vi "processamento_temperatura_velocidade.vi"() -> ()   [LabVIEW 2018]
uses:
  <vilib>/Analysis/NI_AALBase.lvlib
panel:
  in  "Velocidade":path
  out "Velocidade média":dbl format="%0.2f"
  out "Desvio-padrão da temperatura":dbl format="%0.2f"
  out "Temperatura Média":dbl format="%0.2f"
  out "x/y 2":dbl[](array[numeric])
  out "x-y 2":dbl
  out "direito 3":dbl
  out "esquerdo 3":dbl
  in  "Frequência de amostragem - velocidade":dbl
  out "Velocidade":waveform(dbl)(graph)
  out "x/y":dbl[](array[numeric])
  out "x-y":dbl
  out "direito 2":dbl
  out "esquerdo 2":dbl
  in  "Frequência de amostragem - temperatura":dbl
  out "Temperatura":waveform(dbl)(graph)
  in  "stop":bool
  in  "Temperatura":path
  # "PROGRAMA PARA O PROCESSAMENTO CONJUNTO \nDA TEMPERATURA E DA VELOCIDADE"
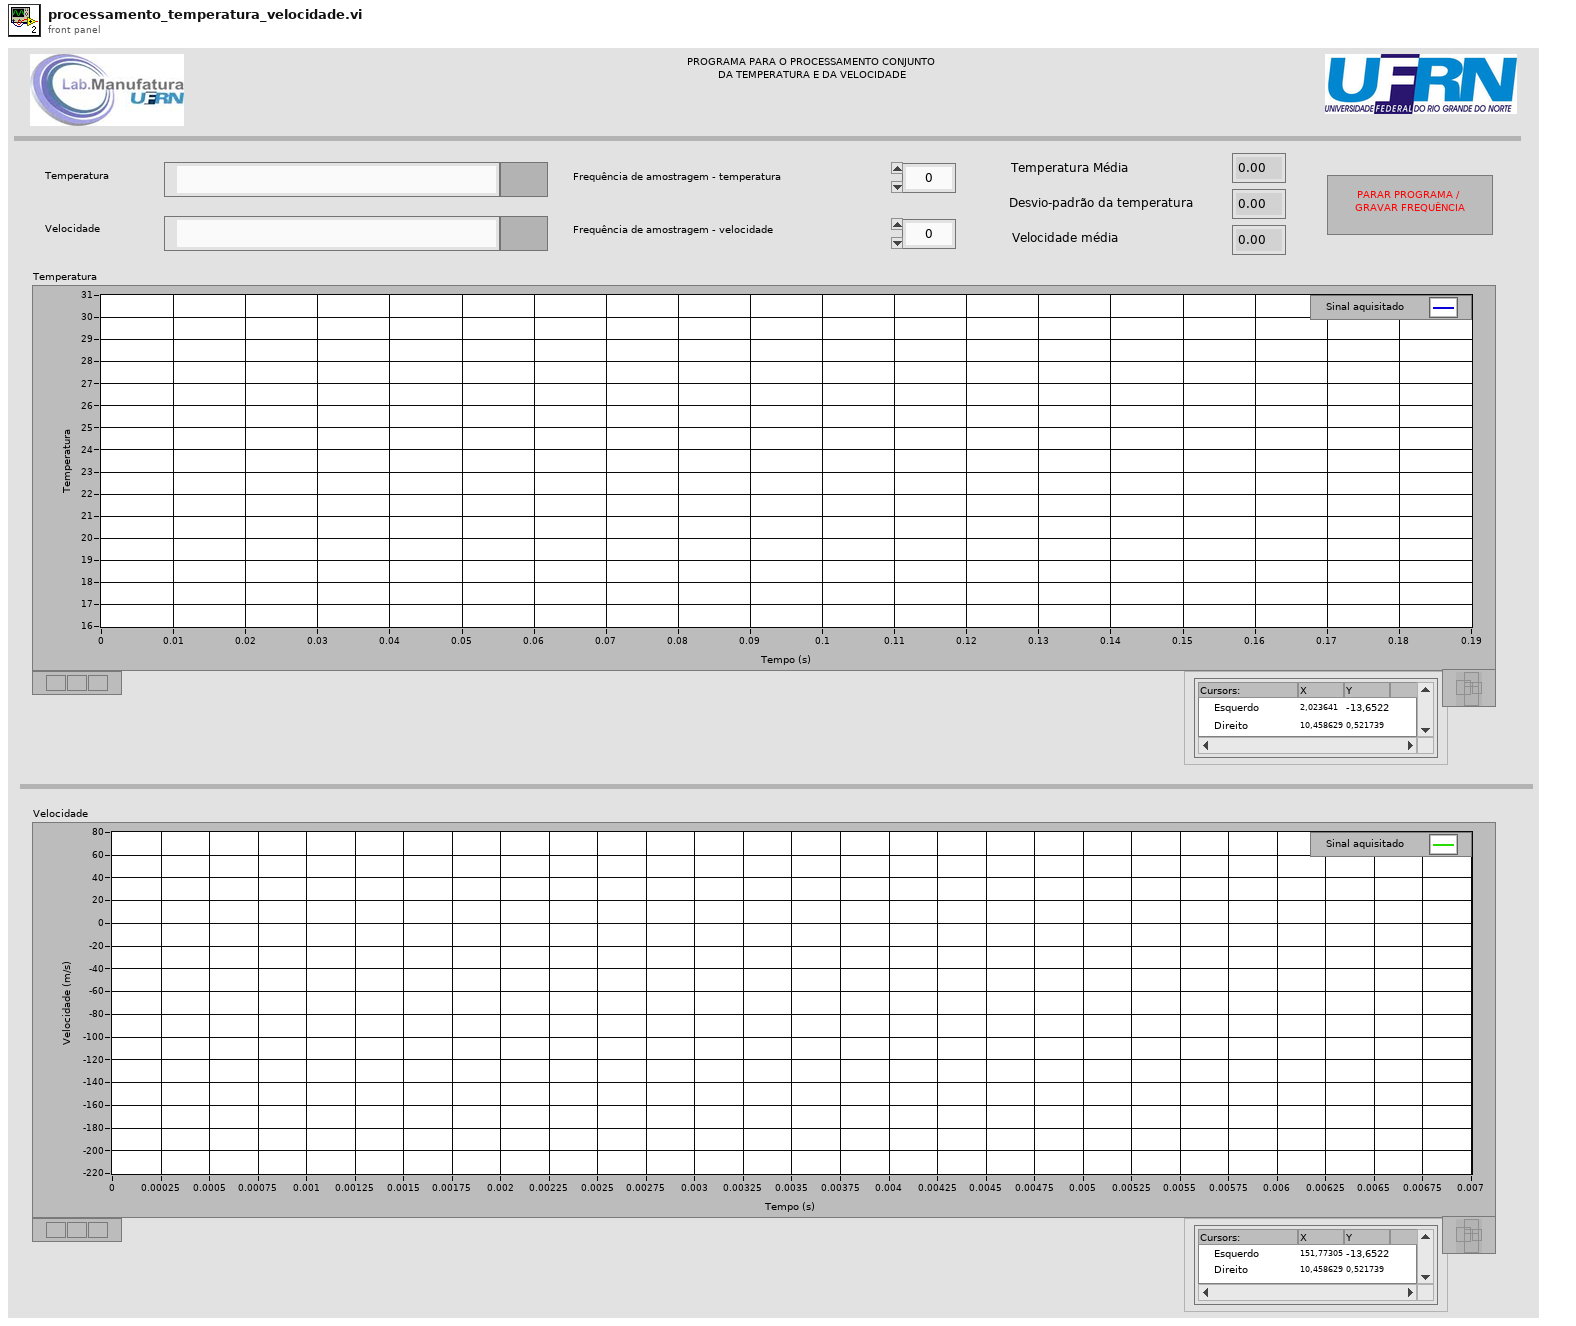
[diagram p1: front panel]
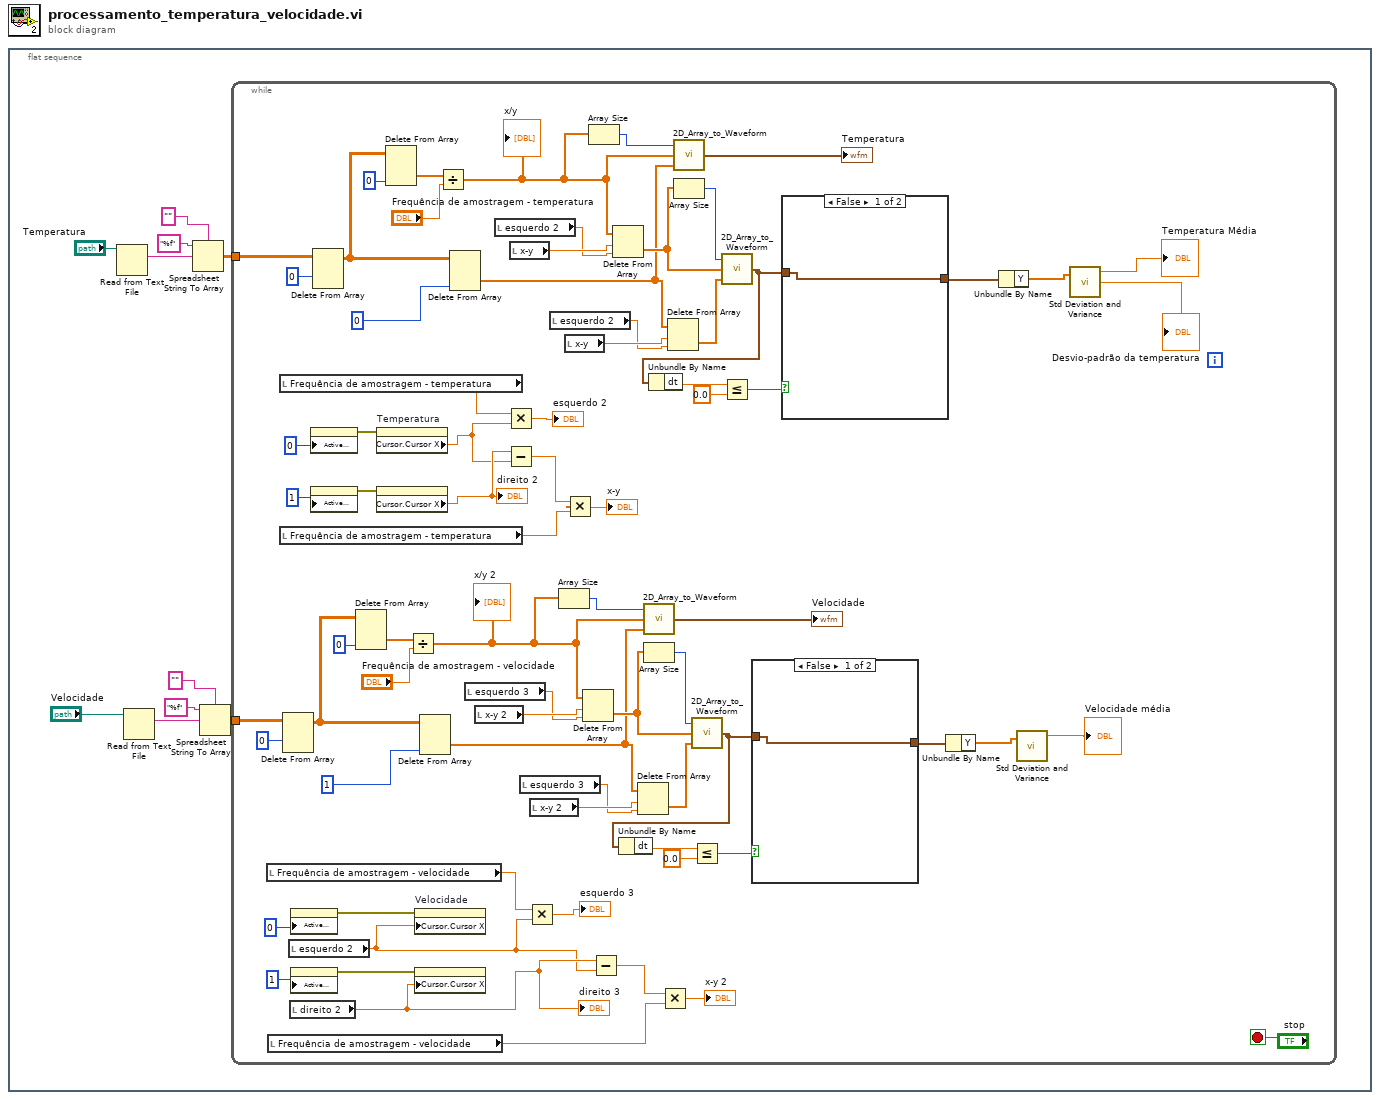
[diagram p0: block diagram]
diagram:
  n1 = flat-sequence {
    frame #0 {
      n2 = Read from Text File(file (use dialog)="Temperatura") -> (text=w7:string)  [unwired: 3 in, 3 out]
      n3 = Read from Text File(file (use dialog)="Velocidade") -> (text=w3:string)  [unwired: 3 in, 3 out]
      n4 = Spreadsheet String To Array(delimiter (Tab)="", format string="%f", spreadsheet string=w7) -> (array=w6:dbl[][])  [unwired: 1 in]
      n5 = Spreadsheet String To Array(delimiter (Tab)="", format string="%f", spreadsheet string=w3) -> (array=w1:dbl[][])  [unwired: 1 in]
      n6 = while {
        tunnel: w6 -> [w21]
        tunnel: w1 -> [w11]
        stop <- "stop" stop-if-true
        n7 = local read "Frequência de amostragem - velocidade"() -> (w31:dbl)
        n8 = local read "Frequência de amostragem - velocidade"() -> (w35:dbl)
        n9 = local read "Frequência de amostragem - temperatura"() -> (w62:dbl)
        n10 = local read "Frequência de amostragem - temperatura"() -> (w66:dbl)
        n11 = Delete From Array(array=w11, index (row)=0) -> (array with subset deleted=w49:dbl[][])  [unwired: 2 in, 1 out]
        n12 = local read "esquerdo 2"() -> (w12:dbl)
        n13 = local read "direito 2"() -> (w13:dbl)
        "direito 3" <- w13
        n14 = property on="Velocidade" class="WFGraph (strict)"("Active Cursor"=u32 0) -> (error out=w44:errorcluster)  [unwired: 2 in, 1 out]
        n15 = property on="Velocidade" class="WFGraph (strict)"("Active Cursor"=u32 1) -> (error out=w43:errorcluster)  [unwired: 2 in, 1 out]
        n16 = property on="Temperatura" class="WFGraph (strict)"("Active Cursor"=u32 0) -> (error out=w76:errorcluster)  [unwired: 2 in, 1 out]
        n17 = property on="Temperatura" class="WFGraph (strict)"("Active Cursor"=u32 1) -> (error out=w75:errorcluster)  [unwired: 2 in, 1 out]
        n18 = Delete From Array(array=w21, index (row)=0) -> (array with subset deleted=w81:dbl[][])  [unwired: 2 in, 1 out]
        n19 = Delete From Array(array=w49, index (col)=0) -> (deleted portion=w48:dbl[])  [unwired: 2 in, 1 out]
        n20 = property on="Temperatura" class="WFGraph (strict)"(error in=w76) -> ("Cursor.Cursor X"=w61:dbl)  [unwired: 1 in, 2 out]
        n21 = property on="Temperatura" class="WFGraph (strict)"(error in=w75) -> ("Cursor.Cursor X"=w74:dbl)  [unwired: 1 in, 2 out]
        "direito 2" <- w74
        n22 = Delete From Array(array=w81, index (col)=0) -> (deleted portion=w80:dbl[])  [unwired: 2 in, 1 out]
        n23 = Divide(x=w48, y="Frequência de amostragem - velocidade") -> (x/y=w29:dbl[])
        "x/y 2" <- w29
        n24 = property on="Velocidade" class="WFGraph (strict)"(error in=w44, "Cursor.Cursor X"=w12) -> ()  [unwired: 1 in, 2 out]
        n25 = property on="Velocidade" class="WFGraph (strict)"(error in=w43, "Cursor.Cursor X"=w13) -> ()  [unwired: 1 in, 2 out]
        n26 = Delete From Array(array=w49, index (col)=1 ("index (row)")) -> (deleted portion=w30:dbl[])  [unwired: 2 in, 1 out]
        n27 = Divide(x=w80, y="Frequência de amostragem - temperatura") -> (x/y=w59:dbl[])
        "x/y" <- w59
        n28 = Delete From Array(array=w81, index (col)=0 ("index (row)")) -> (deleted portion=w60:dbl[])  [unwired: 2 in, 1 out]
        n29 = local read "esquerdo 3"() -> (w38:dbl)
        n30 = local read "x-y 2"() -> (w39:dbl)
        n31 = local read "esquerdo 2"() -> (w69:dbl)
        n32 = Multiply(x=w62, y=w61) -> (x*y=→"esquerdo 2":dbl)
        n33 = Subtract(x=w74, y=w61) -> (x-y=w65:dbl)
        n34 = local read "x-y"() -> (w70:dbl)
        n35 = local read "esquerdo 3"() -> (w36:dbl)
        n36 = Multiply(x=w31, y=w12) -> (x*y=→"esquerdo 3":dbl)
        n37 = local read "x-y 2"() -> (w37:dbl)
        n38 = local read "esquerdo 2"() -> (w67:dbl)
        n39 = Array Size(array=w29) -> (size(s)=w28:i32)
        n40 = local read "x-y"() -> (w68:dbl)
        n41 = Multiply(x=w65, y=w66) -> (x*y=→"x-y":dbl)
        n42 = Delete From Array(array=w29, length=w39, index=w38) -> (deleted portion=w41:dbl[])  [unwired: 1 out]
        n43 = Array Size(array=w59) -> (size(s)=w58:i32)
        n44 = Subtract(x=w13, y=w12) -> (x-y=w34:dbl)
        n45 = Delete From Array(array=w59, length=w70, index=w69) -> (deleted portion=w72:dbl[])  [unwired: 1 out]
        n46 = Delete From Array(array=w30, length=w37, index=w36) -> (deleted portion=w40:dbl[])  [unwired: 1 out]
        n47 = call "2D_Array_to_Waveform.vi"("Y"=w30, "X"=w29, "Nº de amostras"=w28) -> ("output waveform"=→"Velocidade":waveform(dbl))
        n48 = Array Size(array=w41) -> (size(s)=w42:i32)
        n49 = Multiply(x=w34, y=w35) -> (x*y=→"x-y 2":dbl)
        n50 = Delete From Array(array=w60, length=w68, index=w67) -> (deleted portion=w71:dbl[])  [unwired: 1 out]
        n51 = call "2D_Array_to_Waveform.vi"("Y"=w60, "X"=w59, "Nº de amostras"=w58) -> ("output waveform"=→"Temperatura":waveform(dbl))
        n52 = Array Size(array=w72) -> (size(s)=w73:i32)
        n53 = call "2D_Array_to_Waveform.vi"("Y"=w40, "X"=w41, "Nº de amostras"=w42) -> ("output waveform"=w24:waveform(dbl))
        n54 = Unbundle By Name(w24) -> ("dt"=w26:dbl)
        n55 = Less Or Equal?(x=w26, y=0.0) -> (x <= y?=w23:bool)
        n56 = call "2D_Array_to_Waveform.vi"("Y"=w71, "X"=w72, "Nº de amostras"=w73) -> ("output waveform"=w54:waveform(dbl))
        n57 = Unbundle By Name(w54) -> ("dt"=w56:dbl)
        n58 = Less Or Equal?(x=w56, y=0.0) -> (x <= y?=w53:bool)
        n59 = case shown="False" w23 {
          tunnel: w24 -> [w85 _]
          tunnel: [w85 _] -> w14
          frame False {
          }
          frame True {
          }
        }
        n60 = case shown="False" w53 {
          tunnel: w54 -> [w86 _]
          tunnel: [w86 _] -> w20
          frame False {
          }
          frame True {
          }
        }
        n61 = Unbundle By Name(w14) -> ("Y"=w16:dbl[])
        n62 = Unbundle By Name(w20) -> ("Y"=w19:dbl[])
        n63 = call <vilib>:"Std Deviation and Variance.vi"("X"=w16) -> ("mean"=→"Velocidade média":dbl)  [unwired: 1 in, 2 out]
        n64 = call <vilib>:"Std Deviation and Variance.vi"("X"=w19) -> ("mean"=→"Temperatura Média":dbl, "standard deviation"=→"Desvio-padrão da temperatura":dbl)  [unwired: 1 in, 1 out]
      }
    }
  }
